vi "S2DS_ConfigWriteDC (SubVI).vi"(0 "Refnum in":T3, 1 "DAC info list":T1, 3 "error in (no error)":errorcluster) -> (5 "Refnum out":T3, 8 "error out":errorcluster)   [LabVIEW 2025]
uses:
  <vilib>/Utility/config.llb/Config Data RefNum.ctl
  TYPE DEFS/S2DS_DAC info new.ctl
  TYPE DEFS/S2DS_Single DC info.ctl
  <vilib>/Utility/config.llb/Write Key (U32).vi
  <vilib>/Utility/config.llb/Write Key (String).vi
  <vilib>/Utility/config.llb/Write Key (Double).vi
  <vilib>/Utility/config.llb/NI_LVConfig.lvlib
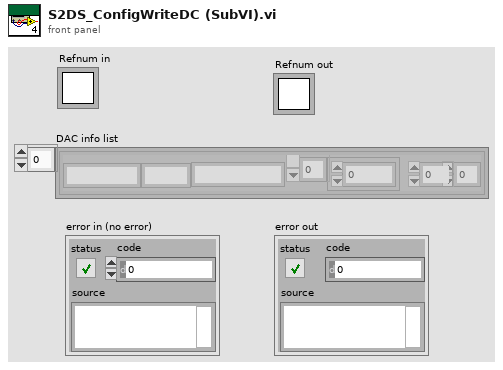
[diagram p1: front panel]
types:
  T1 = typedef "S2DS_DAC info new.ctl" = T2[]
  T2 = typedef "S2DS_Single DC info.ctl" = cluster{"Operation identifier":string, "DC parameters":dbl[], "U":i32, "V":i32, "Name":string, "Unit":string}
  T3 = typedef "NI_LVConfig.lvlib/Config Data RefNum.ctl" = refnum<k1>
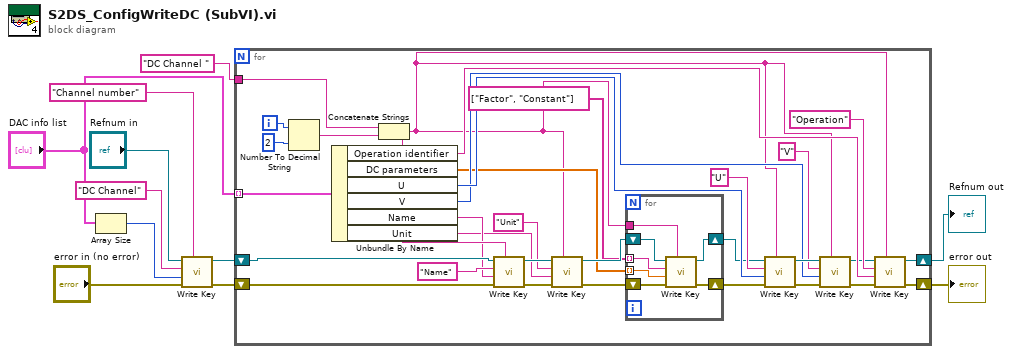
[diagram p0: block diagram]
diagram:
  n1 = Array Size(array="DAC info list") -> (size(s)=w1:i32)
  n2 = call-poly <vilib>:"Write Key.vi"("section"="Channel number", "error in (no error)"="error in (no error)", "value"=w1, "key"="DC Channel", "refnum"="Refnum in") -> ("error out"=w3:errorcluster, "refnum out"=w4:T3)  [unwired: 4 in, 1 out]
  n3 = for {
    tunnel: "DAC info list" -> [w43] mode=indexing
    tunnel: "DC Channel " -> [w39]
    shift-right: [w22] -> w11
    shift-left: w3 -> [w26]
    shift-right: [w21] -> w10
    shift-left: w4 -> [w25]
    i -> [w41]
    n4 = Number To Decimal String(number=w41, width (-)=i16 2) -> (decimal integer string=w38:string)
    n5 = Unbundle By Name(w43) -> ("Operation identifier"=w37:string, "DC parameters"=w18:dbl[], "U"=w36:i32, "V"=w35:i32, "Name"=w13:string, "Unit"=w12:string)
    n6 = Concatenate Strings(w39, w38) -> (w16:string)
    n7 = call-poly <vilib>:"Write Key.vi"("section"=w16, "error in (no error)"=w26, "value"=w13, "key"="Name", "refnum"=w25) -> ("error out"=w28:errorcluster, "refnum out"=w30:T3)  [unwired: 4 in, 1 out]
    n8 = call-poly <vilib>:"Write Key.vi"("section"=w16, "error in (no error)"=w28, "value"=w12, "key"="Unit", "refnum"=w30) -> ("error out"=w27:errorcluster, "refnum out"=w29:T3)  [unwired: 4 in, 1 out]
    n9 = for {
      tunnel: w18 -> [w50] mode=indexing
      tunnel: w16 -> [w49]
      shift-right: [w47] -> w15
      shift-left: w29 -> [w48]
      shift-right: [w45] -> w14
      shift-left: w27 -> [w46]
      tunnel: string[] ["Factor", "Constant"] -> [w44] mode=indexing
      n10 = call-poly <vilib>:"Write Key.vi"("section"=w49, "error in (no error)"=w46, "value"=w50, "key"=w44, "refnum"=w48) -> ("error out"=w45:errorcluster, "refnum out"=w47:T3)  [unwired: 4 in, 1 out]
    }
    n11 = call-poly <vilib>:"Write Key.vi"("section"=w16, "error in (no error)"=w14, "value"=w36, "key"="U", "refnum"=w15) -> ("error out"=w34:errorcluster, "refnum out"=w42:T3)  [unwired: 4 in, 1 out]
    n12 = call-poly <vilib>:"Write Key.vi"("section"=w16, "error in (no error)"=w34, "value"=w35, "key"="V", "refnum"=w42) -> ("error out"=w23:errorcluster, "refnum out"=w24:T3)  [unwired: 4 in, 1 out]
    n13 = call-poly <vilib>:"Write Key.vi"("section"=w16, "error in (no error)"=w23, "value"=w37, "key"="Operation", "refnum"=w24) -> ("error out"=w22:errorcluster, "refnum out"=w21:T3)  [unwired: 4 in, 1 out]
  }
  "error out" <- w11
  "Refnum out" <- w10
